vi "ast_reql_builder.vi"(8 "error in (no error)":errorcluster, 11 "reql":string) -> (0 "error out":errorcluster, 3 "query":refnum<k1>)   [LabVIEW 2017]
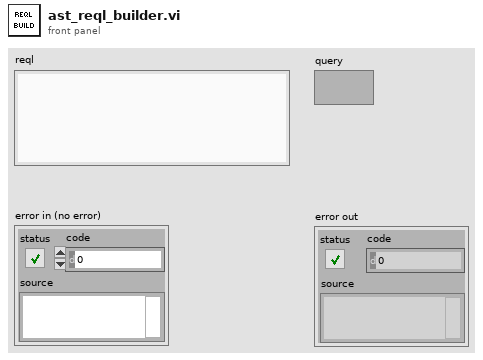
[diagram p1: front panel]
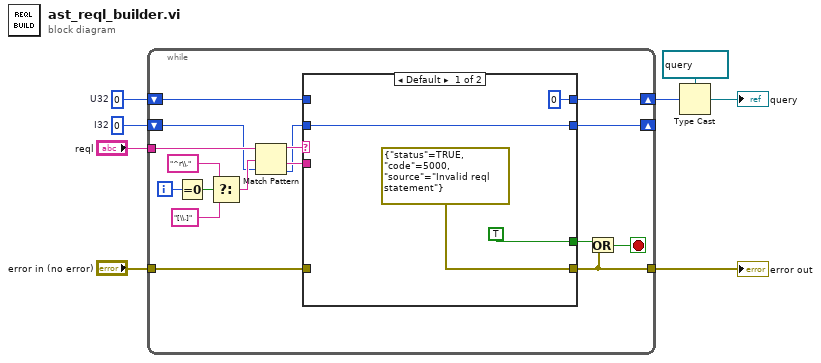
[diagram p0: block diagram]
diagram:
  w1 = 0  # I32
  w2 = u32 0  # U32
  w8 = refnum<k1> refnum items=["query"] ("query out")
  n1 = while {
    tunnel: [w15] -> w6
    tunnel: "error in (no error)" -> [w24]
    tunnel: "reql" -> [w25]
    shift-right: [w13] -> w3
    shift-left: w2 -> [w12]
    shift-right: [w10] -> _
    shift-left: w1 -> [w11]
    i -> [w22]
    stop <- w14 stop-if-true
    n2 = Equal To 0?(x=w22) -> (x = 0?=w21:bool)
    n3 = Select(t="^r\\." ("regular expression"), s=w21, f="[\\.]" ("regular expression")) -> (s? t:f=w18:string)
    n4 = Match Pattern(string=w25, regular expression=w18, offset (0)=w11) -> (before substring=w23:string, after substring=w17:string, offset past match=w9:i32)  [unwired: 1 out]
    n5 = case shown="Default" w23 {
      tunnel: [errorcluster {"status"=TRUE, "code"=5000, "source"="Invalid reql statement"} ("error in (no error)") w32] -> w15
      tunnel: w24 -> [_ w32]
      tunnel: w17 -> [_ _]
      tunnel: [TRUE _] -> w16
      tunnel: [u32 0 ("U32") w31] -> w13
      tunnel: w12 -> [_ w31]
      tunnel: [w26 w30] -> w10
      tunnel: w9 -> [w26 w30]
      frame Default {
      }
      frame "r." {
      }
    }
    n6 = Or(x=w16, y=w15) -> (x .or. y?=w14:bool)
  }
  "error out" <- w6
  n7 = Type Cast(type=w8, x=w3) -> (*(type *) &x=→"query":refnum<k1>)
